vi "Keyence.Main.StatusUpdate.vi"(7 "Idx":i32, 8 "error in":errorcluster, 11 "Data in":T1={"Status"={"State"=enum."Init", "Ref"=refnum, "Bank"=0, "Version"="", "Model"="", "EndTS"=timestamp(0 s since 1904-01-01), "ImgPath"=path ""}, "Sets"={"IP"="192.168.2.1", "Timeout_ms"=5000, "Retries"=0, "ReconnectPeriod_s"=0, "ResetPeriod_s"=0, "ReadImg"=FALSE}, "Code"={"text"="", "status"=FALSE, "corners"=[], "level"=0, "class"="", "path"=path ""}}) -> (0 "error out":errorcluster)   [LabVIEW 2015]
uses:
  Keyence.Data.ctl
  Keyence.Data.Status.ctl
  Keyence.Data.Status.State.ctl
  Keyence.Data.Sets.ctl
  LowLevel/Keyence.CodeDetails.ctl
  LowLevel/Keyence.Global.vi
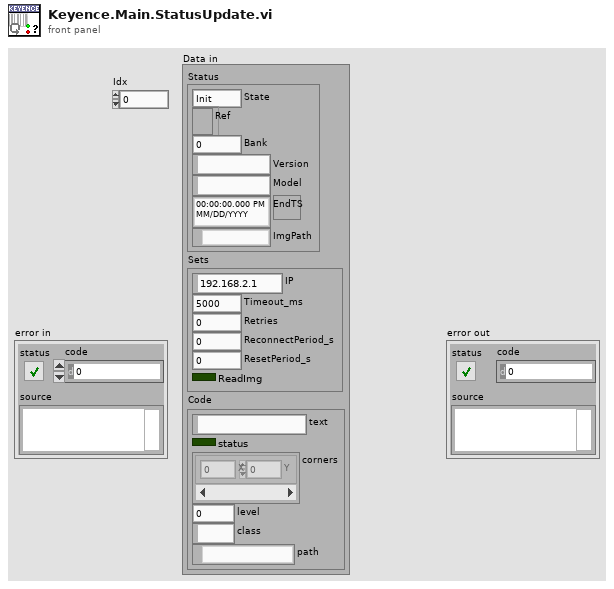
[diagram p1: front panel]
types:
  T1 = typedef "Keyence.Data.ctl" = cluster{"Status":T2, "Sets":T4, "Code":T5}
  T2 = typedef "Keyence.Data.Status.ctl" = cluster{"State":T3, "Ref":refnum<k5>, "Bank":u8, "Version":string, "Model":string, "EndTS":timestamp, "ImgPath":path}
  T3 = typedef "Keyence.Data.Status.State.ctl" = enum16{"First", "Init", "Reset", "Idle", "Scan"}
  T4 = typedef "Keyence.Data.Sets.ctl" = cluster{"IP":string, "Timeout_ms":i32, "Retries":i32, "ReconnectPeriod_s":i32, "ResetPeriod_s":i32, "ReadImg":bool}
  T5 = typedef "Keyence.CodeDetails.ctl" = cluster{"text":string, "status":bool, "corners":cluster{"X":i32, "Y":i32}[], "level":u8, "class":string, "path":path}
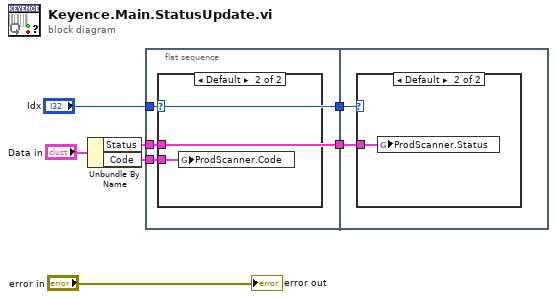
[diagram p0: block diagram]
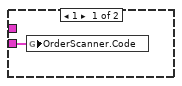
[diagram p2: hidden frame]
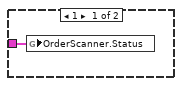
[diagram p3: hidden frame]
diagram:
  n1 = Unbundle By Name("Data in") -> ("Status"=w6:T2, "Code"=w4:T5)
  n2 = flat-sequence {
    tunnel: w6 -> [w8]
    tunnel: w4 -> [w10]
    tunnel: [w9] -> w3
    tunnel: "Idx" -> [w9]
    tunnel: [w8] -> w1
    tunnel: w3 -> [w14]
    tunnel: w1 -> [w13]
    frame #0 {
      n3 = case shown="Default" w9 {
        tunnel: w8 -> [_ _]
        tunnel: w10 -> [w11 w12]
        frame 1 {
          n4 = global write "Keyence.Global.vi" "OrderScanner.Code"(w11) -> ()
        }
        frame Default {
          n5 = global write "Keyence.Global.vi" "ProdScanner.Code"(w12) -> ()
        }
      }
    }
    frame #1 {
      n6 = case shown="Default" w14 {
        tunnel: w13 -> [w15 w16]
        frame 1 {
          n7 = global write "Keyence.Global.vi" "OrderScanner.Status"(w15) -> ()
        }
        frame Default {
          n8 = global write "Keyence.Global.vi" "ProdScanner.Status"(w16) -> ()
        }
      }
    }
  }
  "error out" <- "error in"
